vi "sub_imu-str-2-data.vi"(8 "error in":errorcluster, 11 "read buffer":string) -> (0 "error out":errorcluster, 3 "heading":dbl)   [LabVIEW 2019]
uses:
  Ctrl/cmd_common.ctl
panel:
  out "yaw":dbl
  out "pitch":dbl
  out "roll":dbl
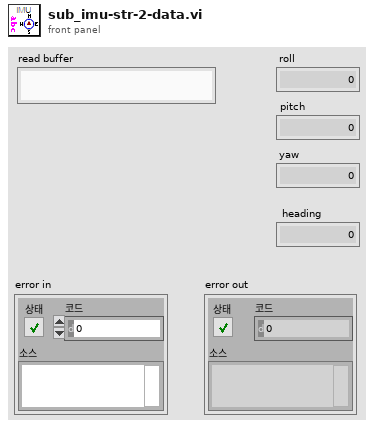
[diagram p1: front panel]
types:
  T1 = typedef "cmd_common.ctl" = enum16{"read", "write"}
  T2 = cluster{"angle":dbl[], "acc":dbl[], "mag":dbl[], "gyr":dbl[]}
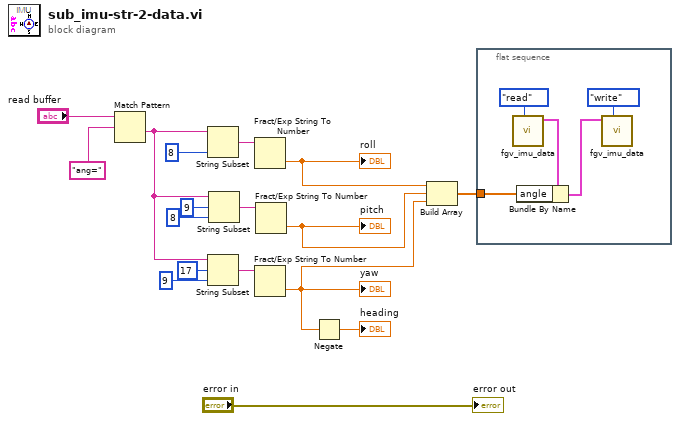
[diagram p0: block diagram]
diagram:
  n1 = Match Pattern(string="read buffer", regular expression="ang=" ("정규식")) -> (after substring=w6:string)  [unwired: 1 in, 3 out]
  n2 = String Subset(string=w6, length (rest)=8 ("길이(나머지)")) -> (substring=w13:string)  [unwired: 1 in]
  n3 = String Subset(string=w6, offset (0)=17 ("오프셋(0)"), length (rest)=9 ("길이(나머지)")) -> (substring=w15:string)
  n4 = String Subset(string=w6, offset (0)=9 ("오프셋(0)"), length (rest)=8 ("길이(나머지)")) -> (substring=w8:string)
  n5 = Fract/Exp String To Number(string=w13) -> (number=w5:dbl)  [unwired: 3 in, 1 out]
  "roll" <- w5
  n6 = Fract/Exp String To Number(string=w15) -> (number=w3:dbl)  [unwired: 3 in, 1 out]
  "yaw" <- w3
  n7 = Fract/Exp String To Number(string=w8) -> (number=w4:dbl)  [unwired: 3 in, 1 out]
  "pitch" <- w4
  n8 = Negate(x=w3) -> (-x=→"heading":dbl)
  n9 = Build Array(w5, w4, w3) -> (w2:dbl[])
  n10 = flat-sequence {
    tunnel: w2 -> [w18]
    frame #0 {
      n11 = call "fgv_imu_data.vi"("cmd"=cmd_common."read") -> ("IMD data out"=w20:T2)  [unwired: 9 in, 1 out]
      n12 = Bundle By Name(cluster=w20, "angle"=w18) -> (w19:T2)
      n13 = call "fgv_imu_data.vi"("cmd"=cmd_common."write", "IMD data"=w19) -> ()  [unwired: 8 in, 2 out]
    }
  }
  "error out" <- "error in"
